vi "Hardware Config - format and values.vi"(11 "Hardware Configuration":T4={"Dev. PC"=FALSE, "Swap XY on stage"=FALSE, "No of AOD"=0, "MC Supported"=FALSE, "Axial MC"=FALSE, "Computer MAC address"="", "Externalise Triggers"=FALSE, "Trigger HW config"={"Available Device List"=0, "Device Address"=""}, "DAQmx Chan"={"Pockels AO"="", "Hard shutter AO"="", "PMT AOs"="", "Galvo AOs"="", "Power meter AI"=""}, "XYZ Stage Control Config"=enum."None", "XY stage available"=FALSE, "XY Comms Config Cluster"={"Name"="", "Device Address"="", "Port "=0, "Baudrate"=0, "Comms Type"=enum."GPIB-IEEE488"}, "Y stage available"=FALSE, "Y Comms Config Cluster"={"Name"="", "Device Address"="", "Port "=0, "Baudrate"=0, "Comms Type"=enum."GPIB-IEEE488"}, "Z stage available"=FALSE, "Z Comms Config Cluster "={"Name"="COM7", "Device Address"="", "Port "=0, "Baudrate"=0, "Comms Type"=enum."GPIB-IEEE488"}, "Encoder available"=FALSE, "Encoder"={"IP address"="224.0.1.103", "Port"=7000, "Wheel radius (cm)"=16.0, "Encoder Trigger"=""}, "VidRec available"=FALSE, "Cam VidRec"={"DO flag-Video record"="", "DO flag-Trial start"=""}, "Laser Power Control HW config"={"Laser Power Control"="", "Laser Power Modulation Control"=enum."NI"}, "Laser 1 available"=FALSE, "Laser 1 config cluster"={"COM port"="COM7", "Baud Rate"=0, "Type"=""}, "Prechirper 1 available"=FALSE, "Prechirper 1 config cluster"={"Type"="", "Baud Rate"=0, "COM port"="COM7"}, "Control system.FPGA available?"=FALSE, "Control Sys. HW config"={"Control system.FPGA Type"=enum."Virtex 5", "Control system.Network adapter name"="", "Control system.MAC address"="", "Control system.Ethernet Port"=0, "Control system.Ethernet Port Opened"=FALSE}, "DAQ FPGA HW Config"={"FGPA Ref"=refnum, "Target"="RIO0", "input card type"=enum."AC Card"}, "PMT Control Voltage Limits"={"Lower Limit"=0.0, "Upper Limit"=0.0}} {"Encoder"."Wheel radius (cm)" format="%#_13g"}) -> (0 "String":string[](array[string]), 1 "String":T1, 2 "Numeric":dbl[](array[numeric]), 3 "Numeric":T3=[{"key"="Encoder.Port", "Save?"=TRUE, "Default"=7000.0}, {"key"="Encoder.Wheel radius (cm)", "Save?"=TRUE, "Default"=16.0}, {"key"="DAQ FPGA.Input type AC/DC", "Save?"=TRUE, "Default"=1.0}, {"key"="Num AOD", "Save?"=TRUE, "Default"=4.0}, {"key"="Trigger.AvailableDeviceList", "Save?"=TRUE, "Default"=1.0}, {"key"="XY Stage.Baudrate", "Save?"=TRUE, "Default"=9600.0}, {"key"="Z Stage.Baudrate", "Save?"=TRUE, "Default"=9600.0}, {"key"="Laser.Baudrate", "Save?"=TRUE, "Default"=19200.0}, {"key"="Prechirper.Baudrate", "Save?"=TRUE, "Default"=115200.0}], 4 "Boolean":bool[](array[boolean]), 6 "Boolean":T2=[{"key"="DevPC - No hardware", "Save?"=TRUE, "Default"=FALSE}, {"key"="MC Supported", "Save?"=TRUE, "Default"=FALSE}, {"key"="Axial MC", "Save?"=TRUE, "Default"=FALSE}, {"key"="Are X Y Swapped", "Save?"=TRUE, "Default"=FALSE}, {"key"="Encoder.Available?", "Save?"=TRUE, "Default"=FALSE}, {"key"="Externalise Triggers", "Save?"=TRUE, "Default"=TRUE}, {"key"="Cam VidRec.Available", "Save?"=TRUE, "Default"=TRUE}, {"key"="Control system.Ctrl FPGA available", "Save?"=TRUE, "Default"=TRUE}, {"key"="XY Stage.Available?", "Save?"=TRUE, "Default"=TRUE}, {"key"="Z Stage.Available?", "Save?"=TRUE, "Default"=FALSE}, {"key"="Laser.Available?", "Save?"=TRUE, "Default"=TRUE}, {"key"="Prechirper.Available", "Save?"=TRUE, "Default"=TRUE}])   [LabVIEW 2020]
uses:
  Typedefs/Hardware Configuration settings.ctl
  Typedefs/Triggers HW config.ctl
  Typedefs/DAQmx physical channels cluster.ctl
  Peripherals Control/XYZ Stage/Control/typedefs/XYZControlConfig.ctl
  Typedefs/Peripherals comms config cluster.ctl
  Typedefs/Comms Type.ctl
  Typedefs/Encoder config cluster.ctl
  Typedefs/Cam VidRec HW config setup cluster.ctl
  Typedefs/Laser Power Control HW config.ctl
  Typedefs/Laser 1 config cluster.ctl
  Typedefs/PreChirper 1 config cluster.ctl
  Typedefs/Control Sys HW config cluster.ctl
  Typedefs/DAQ FPGA HW config cluster.ctl
  RIG-SPECIFIC FILES/FPGA Refs/FPGA Ref.ctl
  <vilib>/userDefined/High Color/nirio_resource_hc.ctl
  Typedefs/FPGA input type AC-DC.ctl
  Typedefs/PMT Control Voltage limits.ctl
  Typedefs/Ini file interface (DBL).ctl
  Typedefs/Ini file interface (Boolean).ctl
  Typedefs/Ini file interface (String).ctl
panel:
  out "Boolean Default cluster":i32
  out "Boolean values":i32
  out "Numeric Values":i32
  out "Numeric Default Cluster":i32
  out "String values":i32
  out "String Default Cluster":i32
  # "Numeric Array Sizes"
  # "String Array Sizes"
  # "Boolean Array Sizes"
  # "(make , model etc)"
  # "(COM Port / IP Address / service address etc.)"
  # "(Port for ethernet / channel for BT)"
  # "(make , model etc)"
  # "(COM Port / IP Address / service address etc.)"
  # "(Port for ethernet / channel for BT)"
  # "(make , model etc)"
  # "(COM Port / IP Address / service address etc.)"
  # "(Port for ethernet / channel for BT)"
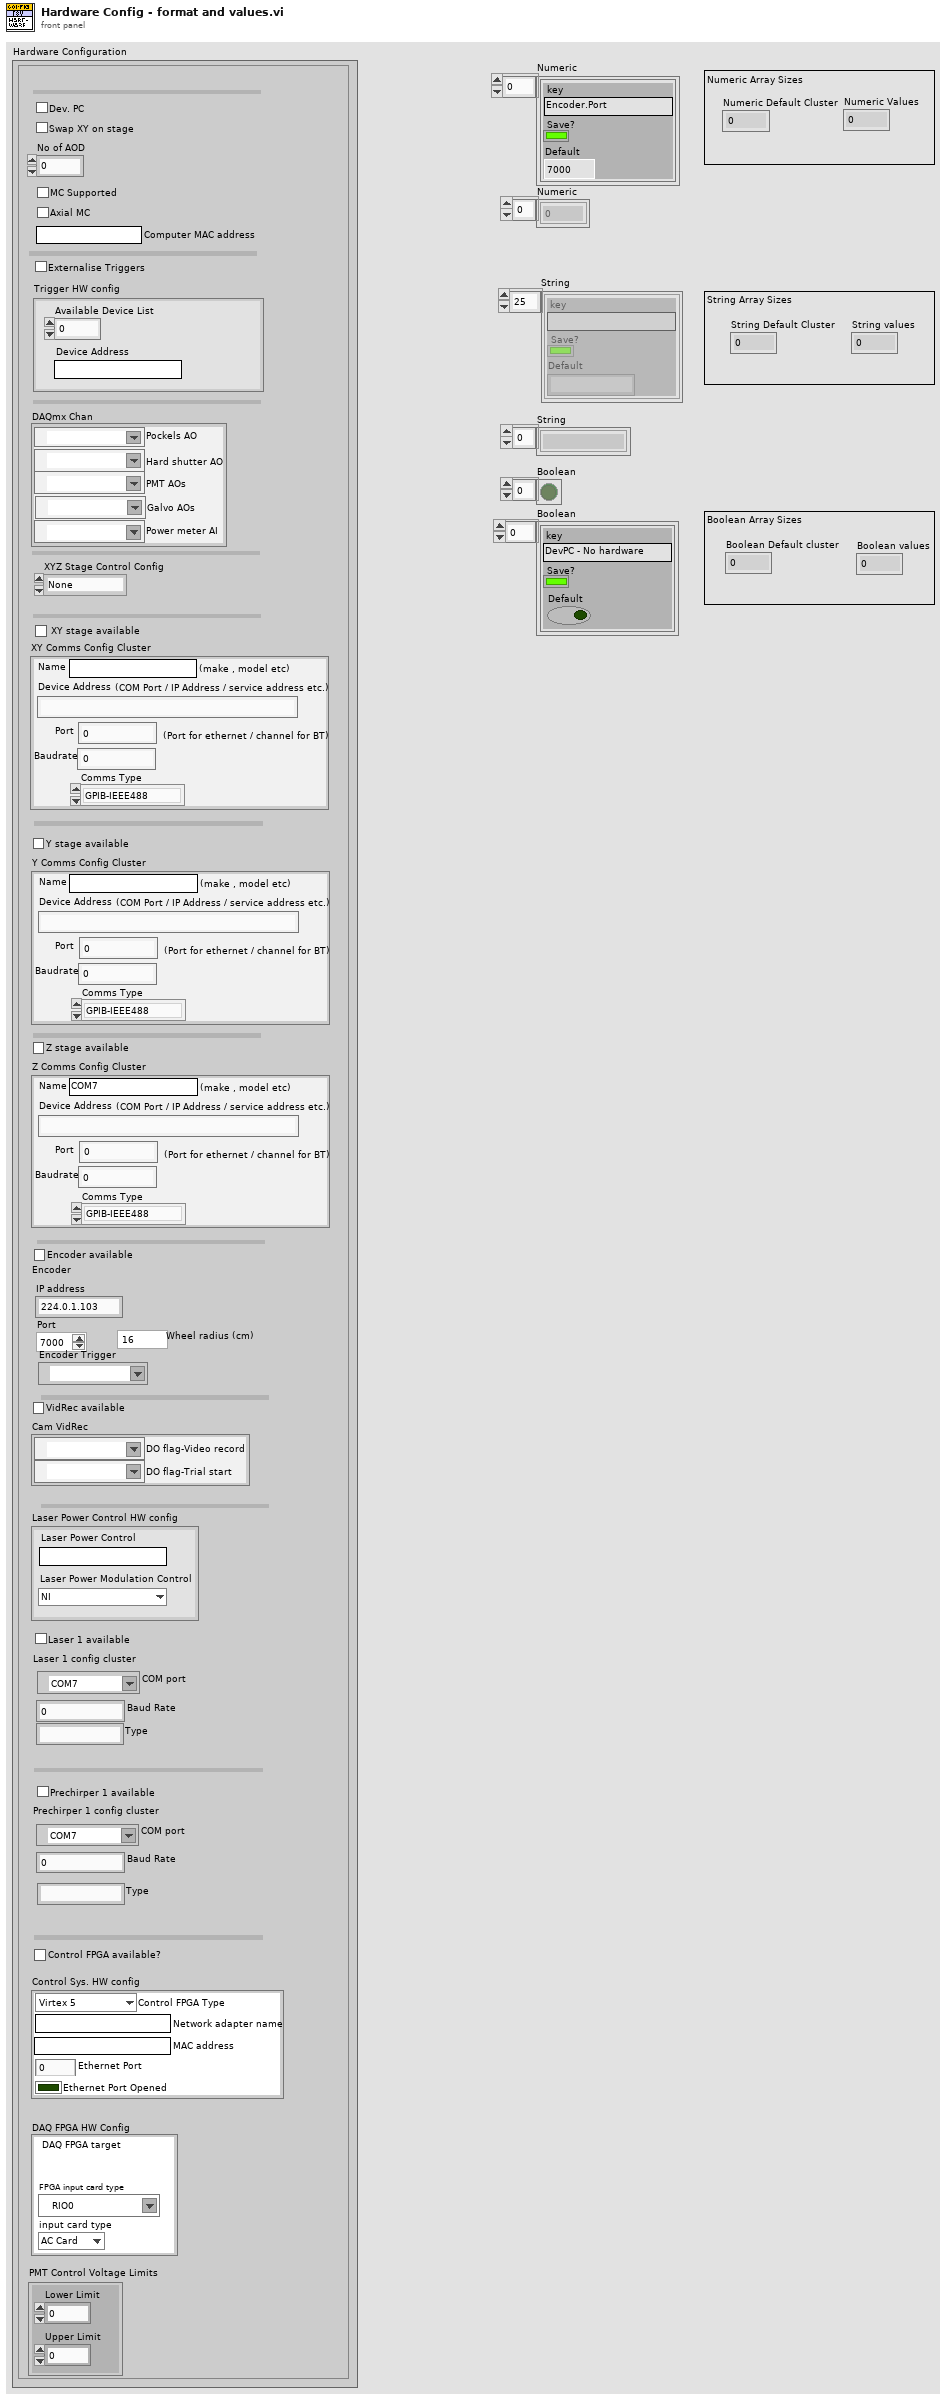
[diagram p1: front panel]
types:
  T1 = typedef "Ini file interface (String).ctl" = cluster{"key":string, "Save?":bool, "Default":string}[]
  T2 = typedef "Ini file interface (Boolean).ctl" = cluster{"key":string, "Save?":bool, "Default":bool}[]
  T3 = typedef "Ini file interface (DBL).ctl" = cluster{"key":string, "Save?":bool, "Default":dbl}[]
  T4 = typedef "Hardware Configuration settings.ctl" = cluster{"Dev. PC":bool, "Swap XY on stage":bool, "No of AOD":u8, "MC Supported":bool, "Axial MC":bool, "Computer MAC address":string, "Externalise Triggers":bool, "Trigger HW config":T5, "DAQmx Chan":T6, "XYZ Stage Control Config":T7, "XY stage available":bool, "XY Comms Config Cluster":T8, "Y stage available":bool, "Y Comms Config Cluster":T8, "Z stage available":bool, "Z Comms Config Cluster ":T8, "Encoder available":bool, "Encoder":T10, "VidRec available":bool, "Cam VidRec":T11, "Laser Power Control HW config":T12, "Laser 1 available":bool, "Laser 1 config cluster":T13, "Prechirper 1 available":bool, "Prechirper 1 config cluster":T14, "Control system.FPGA available?":bool, "Control Sys. HW config":T15, "DAQ FPGA HW Config":T16, "PMT Control Voltage Limits":T20}
  T5 = typedef "Triggers HW config.ctl" = cluster{"Available Device List":i32, "Device Address":string}
  T6 = typedef "DAQmx physical channels cluster.ctl" = cluster{"Pockels AO":tag, "Hard shutter AO":tag, "PMT AOs":tag, "Galvo AOs":tag, "Power meter AI":tag}
  T7 = typedef "XYZControlConfig.ctl" = enum16{"None", "XYZ", "XY-Z", "X-Y-Z", "Z"}
  T8 = typedef "Peripherals comms config cluster.ctl" = cluster{"Name":string, "Device Address":string, "Port ":u16, "Baudrate":i32, "Comms Type":T9}
  T9 = typedef "Comms Type.ctl" = enum16{"GPIB-IEEE488", "Serial-RS232", "Serial-RS485", "Serial-RS422", "Serial-USB", "Ethernet-TCP/IP", "Ethernet-UDP"}
  T10 = typedef "Encoder config cluster.ctl" = cluster{"IP address":string, "Port":u16, "Wheel radius (cm)":dbl, "Encoder Trigger":tag}
  T11 = typedef "Cam VidRec HW config setup cluster.ctl" = cluster{"DO flag-Video record":tag, "DO flag-Trial start":tag}
  T12 = typedef "Laser Power Control HW config.ctl" = cluster{"Laser Power Control":string, "Laser Power Modulation Control":enum16{"NI", "FPGA"}}
  T13 = typedef "Laser 1 config cluster.ctl" = cluster{"COM port":refnum<visa-resource-name>, "Baud Rate":i32, "Type":string}
  T14 = typedef "PreChirper 1 config cluster.ctl" = cluster{"Type":string, "Baud Rate":i32, "COM port":refnum<visa-resource-name>}
  T15 = typedef "Control Sys HW config cluster.ctl" = cluster{"Control system.FPGA Type":enum16{"Virtex 5", "Virtex 7"}, "Control system.Network adapter name":string, "Control system.MAC address":string, "Control system.Ethernet Port":u32, "Control system.Ethernet Port Opened":bool}
  T16 = typedef "DAQ FPGA HW config cluster.ctl" = cluster{"FGPA Ref":T17, "Target":T18, "input card type":T19}
  T17 = typedef "FPGA Ref.ctl" = refnum<k20>
  T18 = typedef "nirio_resource_hc.ctl" = tag
  T19 = typedef "FPGA input type AC-DC.ctl" = enum16{"AC Card", "DC Card"}
  T20 = typedef "PMT Control Voltage limits.ctl" = cluster{"Lower Limit":dbl, "Upper Limit":dbl}
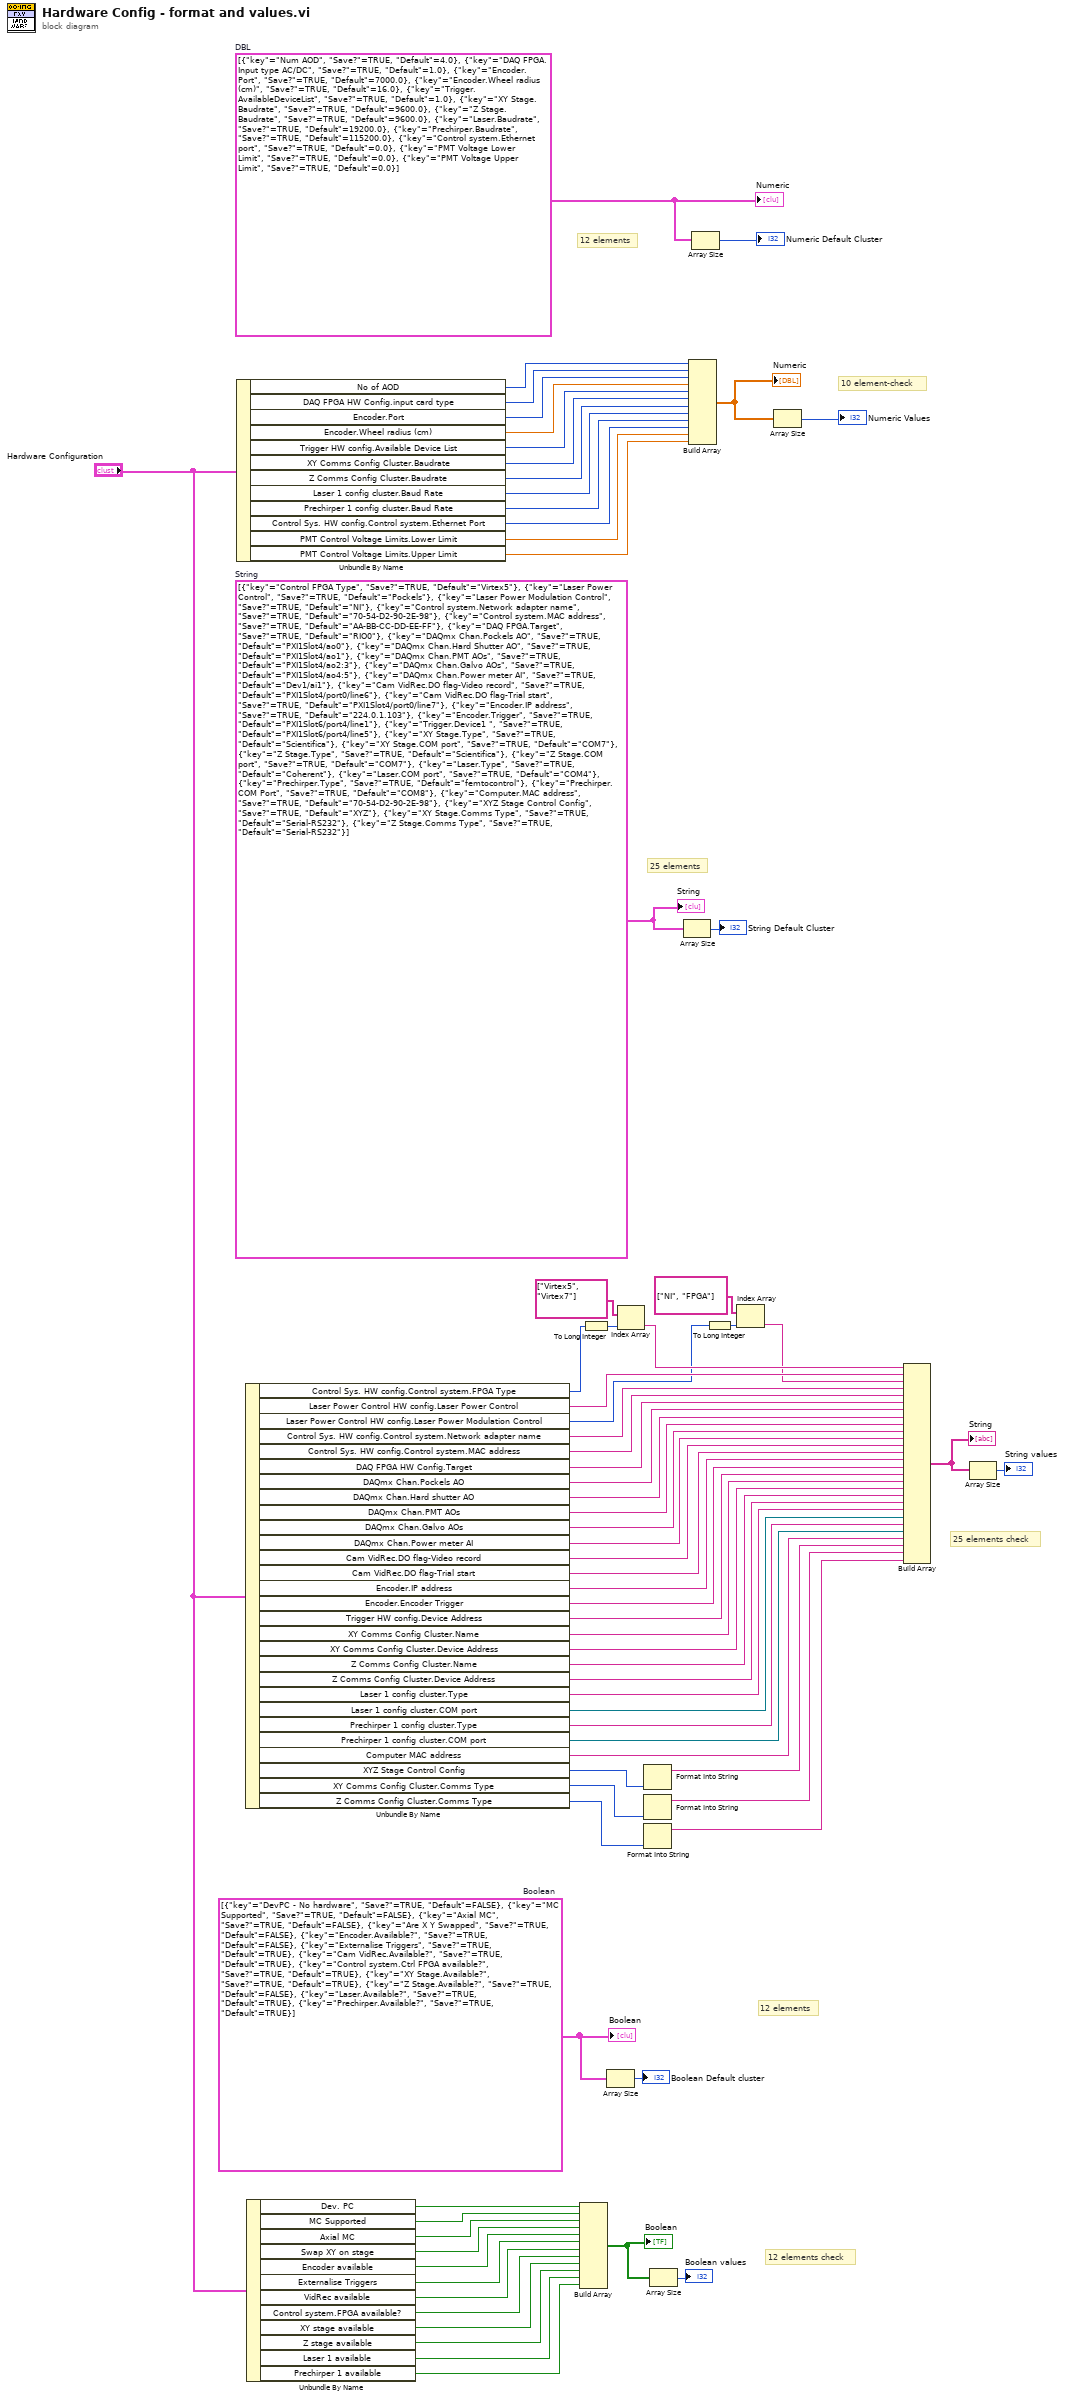
[diagram p0: block diagram]
diagram:
  w20 = T2 [{"key"="DevPC - No hardware", "Save?"=TRUE, "Default"=FALSE}, {"key"="MC Supported", "Save?"=TRUE, "Default"=FALSE}, {"key"="Axial MC", "Save?"=TRUE, "Default"=FALSE}, {"key"="Are X Y Swapped", "Save?"=TRUE, "Default"=FALSE}, {"key"="Encoder.Available?", "Save?"=TRUE, "Default"=FALSE}, {"key"="Externalise Triggers", "Save?"=TRUE, "Default"=TRUE}, {"key"="Cam VidRec.Available?", "Save?"=TRUE, "Default"=TRUE}, {"key"="Control system.Ctrl FPGA available?", "Save?"=TRUE, "Default"=TRUE}, {"key"="XY Stage.Available?", "Save?"=TRUE, "Default"=TRUE}, {"key"="Z Stage.Available?", "Save?"=TRUE, "Default"=FALSE}, {"key"="Laser.Available?", "Save?"=TRUE, "Default"=TRUE}, {"key"="Prechirper.Available?", "Save?"=TRUE, "Default"=TRUE}]  # Boolean
  w30 = T1 [{"key"="Control FPGA Type", "Save?"=TRUE, "Default"="Virtex5"}, {"key"="Laser Power Control", "Save?"=TRUE, "Default"="Pockels"}, {"key"="Laser Power Modulation Control", "Save?"=TRUE, "Default"="NI"}, {"key"="Control system.Network adapter name", "Save?"=TRUE, "Default"="70-54-D2-90-2E-98"}, {"key"="Control system.MAC address", "Save?"=TRUE, "Default"="AA-BB-CC-DD-EE-FF"}, {"key"="DAQ FPGA.Target", "Save?"=TRUE, "Default"="RIO0"}, {"key"="DAQmx Chan.Pockels AO", "Save?"=TRUE, "Default"="PXI1Slot4/ao0"}, {"key"="DAQmx Chan.Hard Shutter AO", "Save?"=TRUE, "Default"="PXI1Slot4/ao1"}, {"key"="DAQmx Chan.PMT AOs", "Save?"=TRUE, "Default"="PXI1Slot4/ao2:3"}, {"key"="DAQmx Chan.Galvo AOs", "Save?"=TRUE, "Default"="PXI1Slot4/ao4:5"}, {"key"="DAQmx Chan.Power meter AI", "Save?"=TRUE, "Default"="Dev1/ai1"}, {"key"="Cam VidRec.DO flag-Video record", "Save?"=TRUE, "Default"="PXI1Slot4/port0/line6"}, {"key"="Cam VidRec.DO flag-Trial start", "Save?"=TRUE, "Default"="PXI1Slot4/port0/line7"}, {"key"="Encoder.IP address", "Save?"=TRUE, "Default"="224.0.1.103"}, {"key"="Encoder.Trigger", "Save?"=TRUE, "Default"="PXI1Slot6/port4/line1"}, {"key"="Trigger.Device1 ", "Save?"=TRUE, "Default"="PXI1Slot6/port4/line5"}, {"key"="XY Stage.Type", "Save?"=TRUE, "Default"="Scientifica"}, {"key"="XY Stage.COM port", "Save?"=TRUE, "Default"="COM7"}, {"key"="Z Stage.Type", "Save?"=TRUE, "Default"="Scientifica"}, {"key"="Z Stage.COM port", "Save?"=TRUE, "Default"="COM7"}, {"key"="Laser.Type", "Save?"=TRUE, "Default"="Coherent"}, {"key"="Laser.COM port", "Save?"=TRUE, "Default"="COM4"}, {"key"="Prechirper.Type", "Save?"=TRUE, "Default"="femtocontrol"}, {"key"="Prechirper.COM Port", "Save?"=TRUE, "Default"="COM8"}, {"key"="Computer.MAC address", "Save?"=TRUE, "Default"="70-54-D2-90-2E-98"}, {"key"="XYZ Stage Control Config", "Save?"=TRUE, "Default"="XYZ"}, {"key"="XY Stage.Comms Type", "Save?"=TRUE, "Default"="Serial-RS232"}, {"key"="Z Stage.Comms Type", "Save?"=TRUE, "Default"="Serial-RS232"}]  # String
  w25 = T3 [{"key"="Num AOD", "Save?"=TRUE, "Default"=4.0}, {"key"="DAQ FPGA.Input type AC/DC", "Save?"=TRUE, "Default"=1.0}, {"key"="Encoder.Port", "Save?"=TRUE, "Default"=7000.0}, {"key"="Encoder.Wheel radius (cm)", "Save?"=TRUE, "Default"=16.0}, {"key"="Trigger.AvailableDeviceList", "Save?"=TRUE, "Default"=1.0}, {"key"="XY Stage.Baudrate", "Save?"=TRUE, "Default"=9600.0}, {"key"="Z Stage.Baudrate", "Save?"=TRUE, "Default"=9600.0}, {"key"="Laser.Baudrate", "Save?"=TRUE, "Default"=19200.0}, {"key"="Prechirper.Baudrate", "Save?"=TRUE, "Default"=115200.0}, {"key"="Control system.Ethernet port", "Save?"=TRUE, "Default"=0.0}, {"key"="PMT Voltage Lower Limit", "Save?"=TRUE, "Default"=0.0}, {"key"="PMT Voltage Upper Limit", "Save?"=TRUE, "Default"=0.0}]  # DBL
  # "12 elements check"
  # "12 elements"
  # "25 elements check"
  # "25 elements"
  # "10 element-check"
  # "12 elements"
  n1 = Unbundle By Name("Hardware Configuration") -> ("No of AOD"=w40:u8, "DAQ FPGA HW Config.input card type"=w39:T19, "Encoder.Port"=w38:u16, "Encoder.Wheel radius (cm)"=w37:dbl, "Trigger HW config.Available Device List"=w36:i32, "XY Comms Config Cluster.Baudrate"=w35:i32, "Z Comms Config Cluster.Baudrate"=w34:i32, "Laser 1 config cluster.Baud Rate"=w33:i32, "Prechirper 1 config cluster.Baud Rate"=w32:i32, "Control Sys. HW config.Control system.Ethernet Port"=w9:u32, "PMT Control Voltage Limits.Lower Limit"=w8:dbl, "PMT Control Voltage Limits.Upper Limit"=w7:dbl)
  n2 = Unbundle By Name("Hardware Configuration") -> ("Control Sys. HW config.Control system.FPGA Type"=w17:enum16{"Virtex 5", "Virtex 7"}, "Laser Power Control HW config.Laser Power Control"=w74:string, "Laser Power Control HW config.Laser Power Modulation Control"=w13:enum16{"NI", "FPGA"}, "Control Sys. HW config.Control system.Network adapter name"=w73:string, "Control Sys. HW config.Control system.MAC address"=w72:string, "DAQ FPGA HW Config.Target"=w41:T18, "DAQmx Chan.Pockels AO"=w71:tag, "DAQmx Chan.Hard shutter AO"=w70:tag, "DAQmx Chan.PMT AOs"=w69:tag, "DAQmx Chan.Galvo AOs"=w31:tag, "DAQmx Chan.Power meter AI"=w68:tag, "Cam VidRec.DO flag-Video record"=w67:tag, "Cam VidRec.DO flag-Trial start"=w66:tag, "Encoder.IP address"=w65:string, "Encoder.Encoder Trigger"=w64:tag, "Trigger HW config.Device Address"=w63:string, "XY Comms Config Cluster.Name"=w62:string, "XY Comms Config Cluster.Device Address"=w61:string, "Z Comms Config Cluster.Name"=w60:string, "Z Comms Config Cluster.Device Address"=w59:string, "Laser 1 config cluster.Type"=w58:string, "Laser 1 config cluster.COM port"=w57:refnum<visa-resource-name>, "Prechirper 1 config cluster.Type"=w56:string, "Prechirper 1 config cluster.COM port"=w55:refnum<visa-resource-name>, "Computer MAC address"=w10:string, "XYZ Stage Control Config"=w6:T7, "XY Comms Config Cluster.Comms Type"=w5:T9, "Z Comms Config Cluster.Comms Type"=w4:T9)
  n3 = Unbundle By Name("Hardware Configuration") -> ("Dev. PC"=w53:bool, "MC Supported"=w52:bool, "Axial MC"=w51:bool, "Swap XY on stage"=w50:bool, "Encoder available"=w49:bool, "Externalise Triggers"=w48:bool, "VidRec available"=w47:bool, "Control system.FPGA available?"=w46:bool, "XY stage available"=w45:bool, "Z stage available"=w44:bool, "Laser 1 available"=w43:bool, "Prechirper 1 available"=w42:bool)
  n4 = Build Array(w53, w52, w51, w50, w49, w48, w47, w46, w45, w44, w43, w42) -> (w19:bool[])
  "Boolean" <- w19
  n5 = To Long Integer(number=w17) -> (32bit integer=w16:i32)
  n6 = Array Size(array=w20) -> (size(s)=→"Boolean Default cluster":i32)
  n7 = Index Array(array=string[] ["Virtex5", "Virtex7"], index=w16) -> (element=w15:string)
  n8 = Format Into String(w6) -> (resulting string=w3:string)  [unwired: 3 in, 1 out]
  n9 = Format Into String(w5) -> (resulting string=w2:string)  [unwired: 3 in, 1 out]
  n10 = Format Into String(w4) -> (resulting string=w1:string)  [unwired: 3 in, 1 out]
  n11 = Array Size(array=w19) -> (size(s)=→"Boolean values":i32)
  n12 = Array Size(array=w30) -> (size(s)=→"String Default Cluster":i32)
  n13 = Build Array(w40, w39, w38, w37, w36, w35, w34, w33, w32, w9, w8, w7) -> (w23:dbl[])
  "Numeric" <- w23
  n14 = Array Size(array=w25) -> (size(s)=→"Numeric Default Cluster":i32)
  n15 = To Long Integer(number=w13) -> (32bit integer=w12:i32)
  n16 = Index Array(array=string[] ["NI", "FPGA"], index=w12) -> (element=w11:string)
  n17 = Array Size(array=w23) -> (size(s)=→"Numeric Values":i32)
  n18 = Build Array(w15, w74, w11, w73, w72, w41, w71, w70, w69, w31, w68, w67, w66, w65, w64, w63, w62, w61, w60, w59, w58, w57, w56, w55, w10, w3, w2, w1) -> (w27:string[])
  "String" <- w27
  n19 = Array Size(array=w27) -> (size(s)=→"String values":i32)
  "Numeric" <- w25
  "Boolean" <- w20
  "String" <- w30
